vi "Cleanup.vi"(8 "error in (no error)":errorcluster, 11 "SB App in":refnum<class "SB App.lvclass">) -> (0 "error out":errorcluster)   [LabVIEW 2020, in "SB App.lvlib" / "SB App.lvclass"]
uses:
  SB App.lvclass
  SB App.lvclass/SB App.ctl
  <vilib>/IlluminatedG/IG OOPanel/OOPanel/Manager/Manager.lvclass
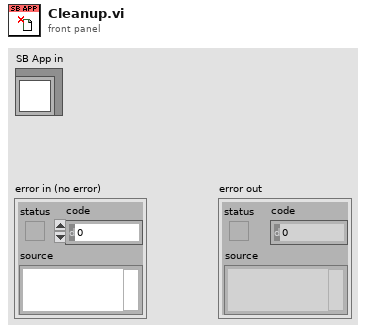
[diagram p1: front panel]
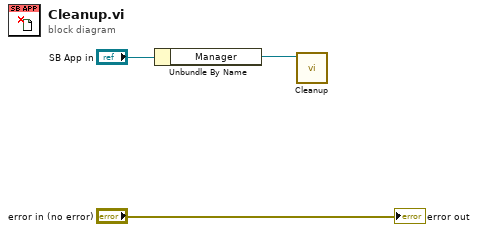
[diagram p0: block diagram]
diagram:
  n1 = Unbundle By Name("SB App in") -> ("Manager"=w1:refnum<class "Manager.lvclass">)
  n2 = call <vilib>:"Cleanup.vi"("Manager in"=w1) -> ()  [unwired: 8 in, 3 out]
  "error out" <- "error in (no error)"
